vi "dvp Vi Get Rgb Gain.vi"(7 "pbGain":sgl, 9 "pgGain":sgl, 10 "prGain":sgl, 11 "handle":u32) -> (1 "pgGain out":sgl, 2 "prGain out":sgl, 3 "function return":u32(ring), 5 "pbGain out":sgl)   [LabVIEW 2018, in "LabViewDVPCamera.lvlib"]
doc: "LabviewDvp2Api dvpStatus dvpViGetRgbGain(dvpHandle handle, float *prGain, float *pgGain, float *pbGain);"
uses:
  LabViewDVPCamera.lvlib
  LabViewDVPCamera/LabViewDVPCamera.dll
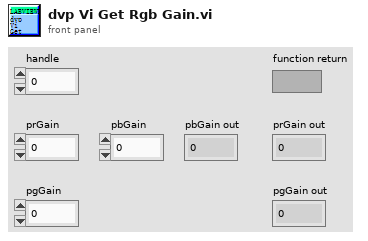
[diagram p1: front panel]
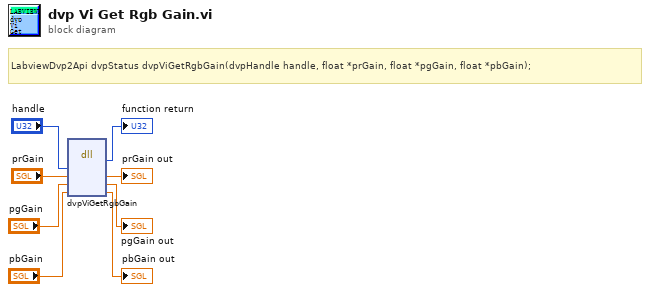
[diagram p0: block diagram]
diagram:
  # "LabviewDvp2Api dvpStatus dvpViGetRgbGain(dvpHandle handle, float *prGain, float *pgGain, float *pbGain);"
  n1 = dll-call lib="C:/Program Files (x86)/DVP2 Labview cn 64/Sample/LabViewDVPCamera/LabViewDVPCamera.*" fn="dvpViGetRgbGain"("handle"="handle", "prGain"="prGain", "pgGain"="pgGain", "pbGain"="pbGain") -> (→"function return":u32, "prGain"=→"prGain out":sgl, "pgGain"=→"pgGain out":sgl, "pbGain"=→"pbGain out":sgl)  [unwired: 4 in, 2 out]
